vi "Do.vi"(8 "error in (no error)":errorcluster, 10 "Actor in":refnum<class "Actor.lvclass">, 11 "DNL_Message Template":refnum<class "Panel Request Msg.lvclass">) -> (0 "error out":errorcluster, 2 "Actor out":refnum<class "Actor.lvclass">)   [LabVIEW 2015, in "EditPanel API.lvlib" / "Panel Request Msg.lvclass"]
doc: "This VI delivers the message to the actor by calling the appropriate method(s) on the actor."
uses:
  Panel Request Msg.lvclass
  <vilib>/ActorFramework/Actor/Actor.lvclass
  Console/Console.lvclass
  Panel Request Msg.lvclass/Panel Request Msg.ctl
  Console/Console.lvclass/Console.ctl
  Console Reply/Console Reply Error Report/Console Reply Error Report.lvclass
  Console Reply/Console Reply/Console Reply.lvclass
  Panel Control_Interface/Panel_interface/Panel Controller Interface.lvclass
  Panle Requeset Behavior/Panel Behavior.lvclass
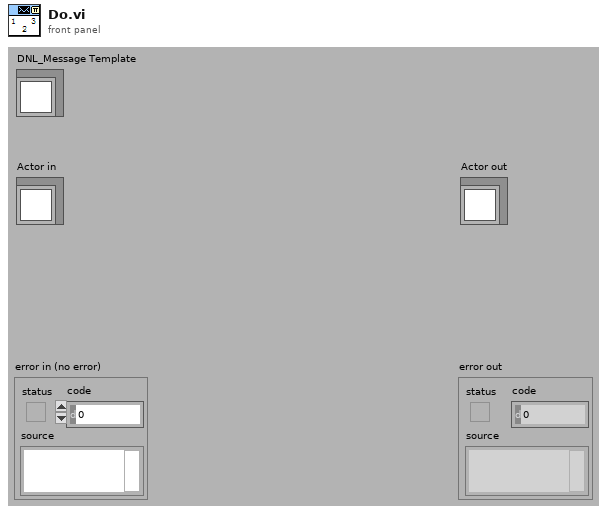
[diagram p1: front panel]
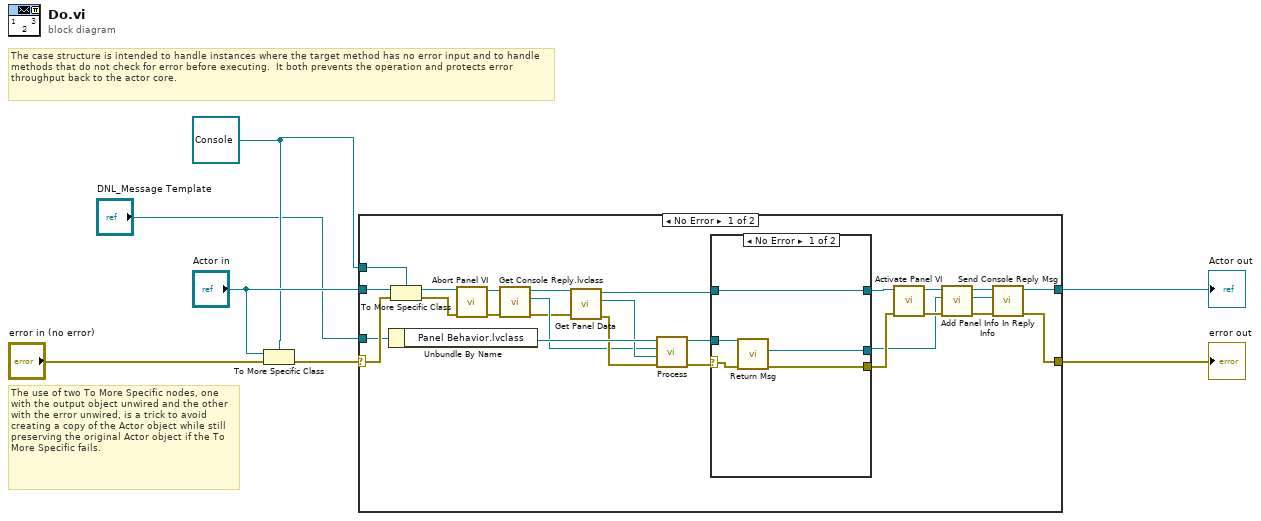
[diagram p0: block diagram]
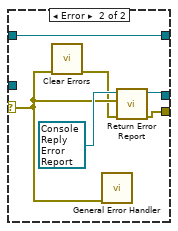
[diagram p2: hidden frame]
diagram:
  w2 = refnum<class "Console.lvclass"> refnum ("Actor in")
  # "The use of two To More Specific nodes, one with the output object unwired and the other with the error unwired, is a trick to avoid creating a copy of the Actor object while still preserving the original Actor object if the To More Specific fails."
  # "The case structure is intended to handle instances where the target method has no error input and to handle methods that do not check for error before executing.  It both prevents the operation and protects error throughput back to the actor core."
  n1 = To More Specific Class(target class=w2, reference="Actor in", error in="error in (no error)") -> (error out=w6:errorcluster)  [unwired: 1 out]
  n2 = case shown="No Error" w6 {
    selector: w6 -> [w31 w47]
    tunnel: [w17 w47] -> w5
    tunnel: [w18 w46] -> w4
    tunnel: "Actor in" -> [w34 w46]
    tunnel: w2 -> [w33 _]
    tunnel: "DNL_Message Template" -> [w27 _]
    frame No Error {
      n3 = Unbundle By Name(w27) -> ("Panel Behavior.lvclass"=w26:refnum<class "Panel Behavior.lvclass">)
      n4 = To More Specific Class(target class=w33, reference=w34, error in=w31) -> (specific class reference=w32:refnum<class "Console.lvclass">, error out=w30:errorcluster)
      n5 = call "Abort Panel VI.vi"("error in (no error)"=w30, "Console in"=w32) -> ("error out"=w11:errorcluster, "Console out"=w12:refnum<class "Console.lvclass">)  [unwired: 8 in]
      n6 = call "Get Console Reply.lvclass.vi"("error in (no error)"=w11, "Console in"=w12) -> ("error out"=w8:errorcluster, "EditPanel API.lvlib:Console Reply.lvclass"=w9:refnum<class "Console Reply.lvclass">, "Console out"=w10:refnum<class "Console.lvclass">)  [unwired: 7 in]
      n7 = call "Get Panel Data.vi"("error in (no error)"=w8, "Console in"=w10) -> ("error out"=w15:errorcluster, "Panel"=w14:refnum<class "Panel Controller Interface.lvclass">, "Console out"=w16:refnum<class "Console.lvclass">)  [unwired: 7 in]
      n8 = call-dynamic "Process.vi"("error in (no error)"=w15, "Panel"=w14, "Console Reply.lvclass"=w9, "Panel Behavior.lvclass"=w26) -> ("error out"=w25:errorcluster, "Panel Behavior.lvclass"=w24:refnum<class "Panel Behavior.lvclass">)  [unwired: 6 in]
      n9 = case shown="No Error" w25 {
        selector: w25 -> [w38 w43]
        tunnel: w16 -> [w37 w45]
        tunnel: [w35 w40] -> w28
        tunnel: [w36 w41] -> w21
        tunnel: [w37 w45] -> w29
        tunnel: w24 -> [w39 _]
        frame No Error {
          n10 = call-dynamic "Return Msg.vi"("error in (no error)"=w38, "Panel Behavior.lvclass"=w39) -> ("error out"=w35:errorcluster, "Console2API Q.lvclass"=w36:refnum<class "Console Reply.lvclass">)  [unwired: 7 in, 1 out]
        }
        frame Error {
          n11 = call <vilib>:"Clear Errors.vi"("error in (no error)"=w43) -> ("error out"=w42:errorcluster)  [unwired: 5 in, 1 out]
          n12 = call <vilib>:"General Error Handler.vi"("error in (no error)"=w43) -> ()  [unwired: 10 in, 5 out]
          n13 = call "Return Error Report.vi"("error in (no error)"=w42, "error Source(No Error)"=w43, "Console Error(Console2API) in"=refnum<class "Console Reply Error Report.lvclass"> refnum) -> ("error out"=w40:errorcluster, "Console Error(Console2API) out"=w41:refnum<class "Console Reply Error Report.lvclass">)  [unwired: 7 in]
        }
      }
      n14 = call "Activate Panel VI.vi"("error in (no error)"=w28, "Console in"=w29) -> ("error out"=w22:errorcluster, "Console out"=w23:refnum<class "Console.lvclass">)  [unwired: 8 in]
      n15 = call "Add Panel Info In Reply Info.vi"("error in (no error)"=w22, "Reply"=w21, "Console in"=w23) -> ("error out"=w19:errorcluster, "Console2API Q out"=w13:refnum<class "Console Reply.lvclass">, "Console out"=w20:refnum<class "Console.lvclass">)  [unwired: 6 in]
      n16 = call "Send Console Reply Msg.vi"("error in (no error)"=w19, "Console Reply"=w13, "Console in"=w20) -> ("error out"=w17:errorcluster, "Console out"=w18:refnum<class "Console.lvclass">)  [unwired: 7 in]
    }
    frame Error {
      # "If type check fails, pass the original object out again."
    }
  }
  "error out" <- w5
  "Actor out" <- w4
